vi "SimpleMotorFF_New.vi"(9 "Ka":dbl, 10 "Kv":dbl, 11 "Ks":dbl) -> (3 "SIMPLE_MOTOR_FF":T1 {"Ka" format="%13.4f"; "Kv" format="%13.4f"; "Ks" format="%13.4f"})   [LabVIEW 2019, in "Trajectory_Library.lvlib"]
doc: "Creates a new SimpleMotorFeedforward with the specified gains. Units of the gain values will dictate units of the computed feedforward. (Generally units should be in meters to match other internal routines.)\n\nThese can be obtained by using the FRC Characterization routine to test your robot.\n\nParameters\n - ks - The static gain. (volts)\n - kv - The velocity gain. (volts seconds/meter)\n - ka - The acceleration gain. (volts seconds^2 / meter )"
uses:
  Trajectory_Library.lvlib
  SIMPLE_MOTOR_FF.ctl
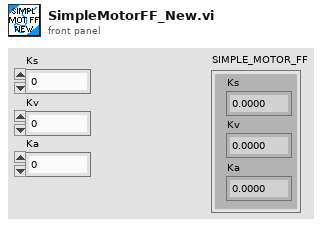
[diagram p1: front panel]
types:
  T1 = typedef "Trajectory_Library.lvlib/SIMPLE_MOTOR_FF.ctl" = cluster{"Ks":dbl, "Kv":dbl, "Ka":dbl}
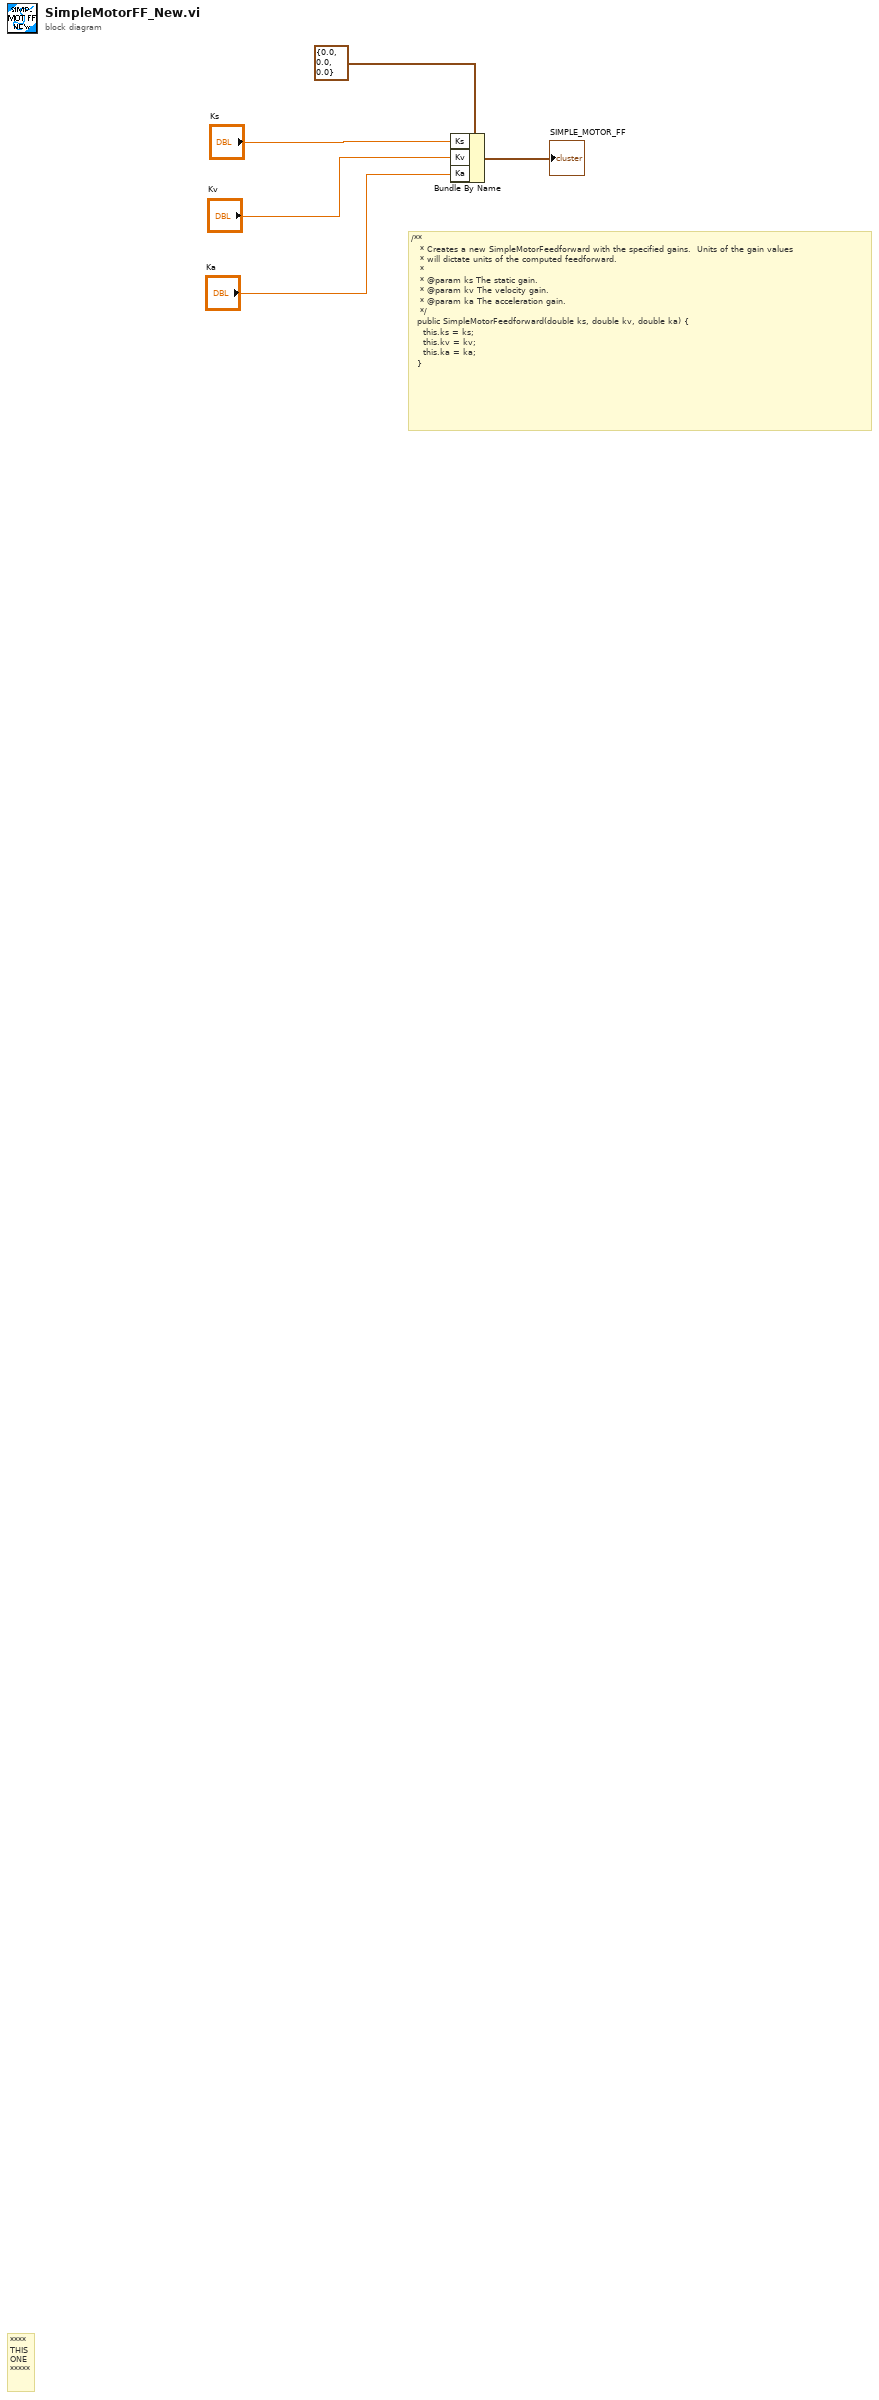
[diagram p0: block diagram]
diagram:
  # "/**\n   * Creates a new SimpleMotorFeedforward with the specified gains.  Units of the gain values\n   * will dictate units of the computed feedforward.\n   *\n   * @param ks The static gain.\n   * @param kv The velocity gain.\n   * @param ka The acceleration gain.\n   */\n  public SimpleMotorFeedforward(double ks, double kv, double ka) {\n    this.ks = ks;\n    this.kv = kv;\n    this.ka = ka;\n  }"
  # "****\nTHIS\nONE\n*****"
  n1 = Bundle By Name(cluster=T1 {"Ks"=0.0, "Kv"=0.0, "Ka"=0.0} ("SIMPLE_MOTOR_FF"), "Ks"="Ks", "Kv"="Kv", "Ka"="Ka") -> (→"SIMPLE_MOTOR_FF":T1)
